vi ".NET Refnum Probe.vi"(1 ".NET Object":refnum<k24>) -> (0 "Stop?":bool)   [LabVIEW 2017]
doc: "Displays the result of calling the ToString() method on the object represented by the .NET refnum, the type of the object, the hash code of the object, and the hex value of the reference.You can use this probe to set a breakpoint if the value is an invalid refnum."
panel:
  out "Display string":string
  in  "Pause if Not a Refnum":bool
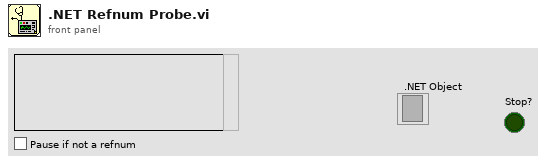
[diagram p1: front panel]
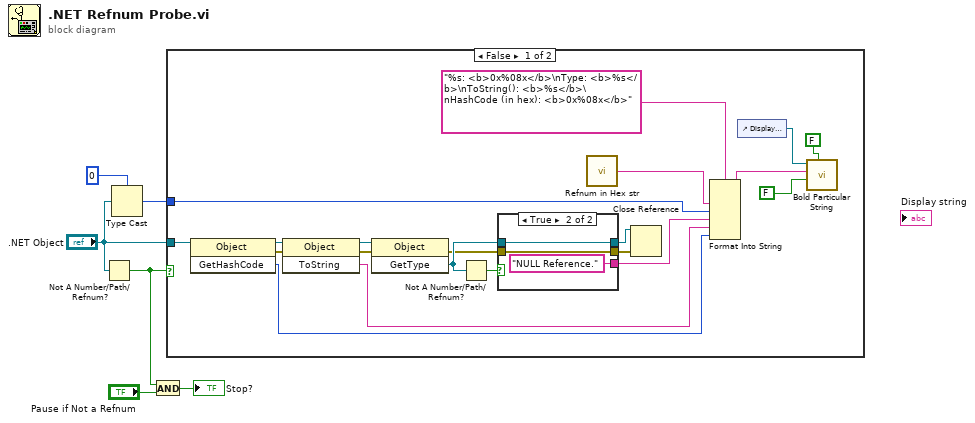
[diagram p0: block diagram]
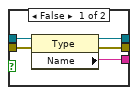
[diagram p2: hidden frame]
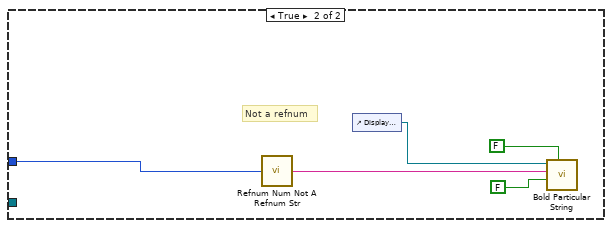
[diagram p3: hidden frame]
diagram:
  n1 = Not A Number/Path/Refnum?(number/path/refnum=".NET Object") -> (NaN/Path/Refnum?=w4:bool)
  n2 = Type Cast(type=u32 0, x=".NET Object") -> (*(type *) &x=w2:u32)
  n3 = And(x=w4, y="Pause if Not a Refnum") -> (x .and. y?=→"Stop?":bool)
  n4 = case shown="False" w4 {
    tunnel: w2 -> [w20 w36]
    tunnel: ".NET Object" -> [w10 _]
    frame False {
      n5 = invoke class="Object" method="GetHashCode"(reference=w10) -> (reference out=w12:refnum<k24>, error out=w11:errorcluster, "GetHashCode"=w9:i32)  [unwired: 2 in]
      n6 = invoke class="Object" method="ToString"(reference=w12, error in=w11) -> (reference out=w14:refnum<k24>, error out=w13:errorcluster, "ToString"=w7:string)  [unwired: 1 in]
      n7 = invoke class="Object" method="GetType"(reference=w14, error in=w13) -> (error out=w15:errorcluster, "GetType"=w18:refnum<k24>)  [unwired: 1 in, 1 out]
      n8 = Not A Number/Path/Refnum?(number/path/refnum=w18) -> (NaN/Path/Refnum?=w19:bool)
      n9 = case shown="True" w19 {
        tunnel: w15 -> [w31 w33]
        tunnel: [w30 "NULL Reference." ("Name")] -> w8
        tunnel: [w29 w33] -> w16
        tunnel: [w28 w34] -> w17
        tunnel: w18 -> [w27 w34]
        frame False {
          n10 = property class="Type"(reference=w27, error in=w31) -> (reference out=w28:refnum<k24>, error out=w29:errorcluster, "Name"=w30:string)
        }
        frame True {
        }
      }
      n11 = call <vilib>:"Refnum in Hex str.vi"() -> ("refnum in hex"=w21:string)
      n12 = Close Reference(reference=w17, error in (no error)=w16) -> ()  [unwired: 1 out]
      n13 = Format Into String(format string="%s: <b>0x%08x</b>\nType: <b>%s</b>\nToString(): <b>%s</b>\nHashCode (in hex): <b>0x%08x</b>", w21, w20, w8, w7, w9) -> (resulting string=w24:string)  [unwired: 2 in, 1 out]
      n14 = control-ref of="Display string"() -> (w26:refnum<vi>)
      n15 = call <vilib>:"Bold Particular String.vi"("Always Refresh? (TRUE)"=FALSE ("Always Refresh? (FALSE)"), "resize string? (TRUE)"=FALSE ("resize string?"), "text to display"=w24, "string refnum"=w26) -> ()  [unwired: 6 in, 2 out]
    }
    frame True {
      # "Not a refnum"
      n16 = call <vilib>:"Refnum Num Not A Refnum Str.vi"("Numeric"=w36) -> ("text to display"=w35:string)
      n17 = control-ref of="Display string"() -> (w38:refnum<vi>)
      n18 = call <vilib>:"Bold Particular String.vi"("Always Refresh? (TRUE)"=FALSE ("Always Refresh? (FALSE)"), "resize string? (TRUE)"=FALSE, "text to display"=w35, "string refnum"=w38) -> ()  [unwired: 6 in, 2 out]
    }
  }
